vi "Update from Process.vi"(8 "error in (no error)":errorcluster, 10 "Value":dbl, 11 "Process State in":refnum<class "Process State.lvclass">) -> (0 "error out":errorcluster, 3 "Process State out":refnum<class "State Actor.lvclass">)   [LabVIEW 2025, in "Process States.lvlib" / "Process State.lvclass"]
doc: "This method defines the default behavior when the actor receives a data point from its Process Actor. The default behavior is to send a Log Event message to the UI with a text string containing the value as its payload."
uses:
  Process State.lvclass
  <vilib>/ni/Actors/State Actor/State Actor/State Actor.lvclass
  <vilib>/ActorFramework/Actor/Actor.lvclass/Actor.ctl
  State Pattern UI/Log Event Msg/Log Event Msg.lvclass/Log Event Msg.ctl
  <vilib>/ActorFramework/Message Enqueuer/Message Enqueuer.lvclass/Message Enqueuer.ctl
  <vilib>/ActorFramework/Message Enqueuer/Enqueue.vi
  State Pattern UI/Log Event Msg/Log Event Msg.lvclass
  <vilib>/ActorFramework/Message Priority Queue/Priority Enqueue.vi
  Process State.lvclass/Process State.ctl
  <vilib>/ActorFramework/Actor/Actor.lvclass
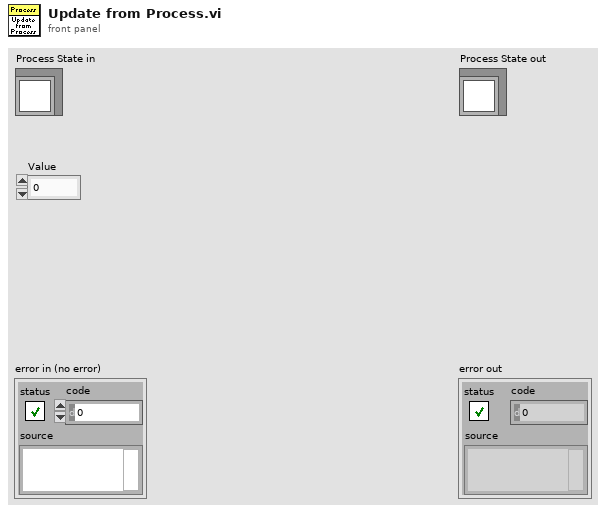
[diagram p1: front panel]
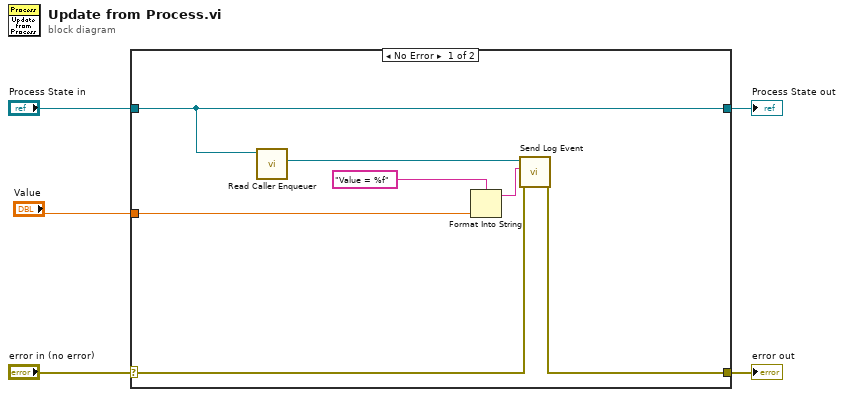
[diagram p0: block diagram]
diagram:
  n1 = case shown="No Error" "error in (no error)" {
    selector: "error in (no error)" -> [w8 w14]
    tunnel: [w7 w14] -> w4
    tunnel: [w9 w13] -> w2
    tunnel: "Process State in" -> [w9 w13]
    tunnel: "Value" -> [w6 _]
    frame No Error {
      n2 = call <vilib>:"Read Caller Enqueuer.vi"("Actor"=w9) -> ("Caller Enqueuer"=w12:refnum<class "Message Enqueuer.lvclass">)  [unwired: 10 in]
      n3 = Format Into String(format string="Value = %f", w6) -> (resulting string=w11:string)  [unwired: 2 in, 1 out]
      n4 = call "Send Log Event.vi"("error in (no error)"=w8, "Event Text"=w11, "Message Enqueuer"=w12) -> ("error out"=w7:errorcluster)  [unwired: 8 in]
    }
    frame Error {
    }
  }
  "error out" <- w4
  "Process State out" <- w2
